vi "SetChannelStatus.vi"(8 "error in (no error)":errorcluster, 10 "Channel Status":string, 11 "Waveform in":waveform(sgl)) -> (0 "error out":errorcluster, 3 "Waveform out":waveform(sgl))   [LabVIEW 2017, in "ChannelStatus.lvlib"]
uses:
  <vilib>/addons/InsightCM/Utilities/ChannelStatus/ChannelStatus.lvlib
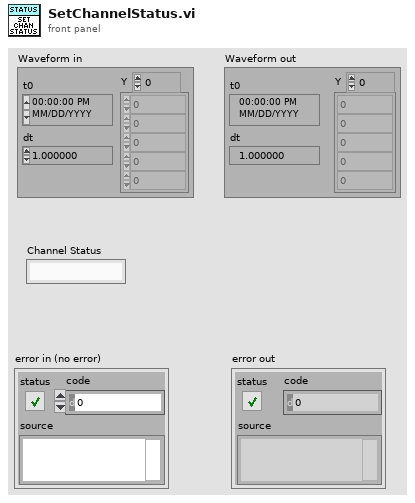
[diagram p1: front panel]
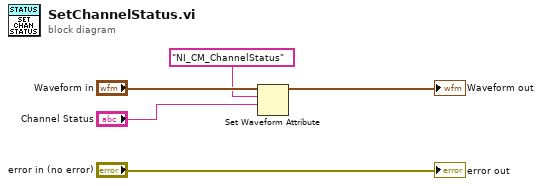
[diagram p0: block diagram]
diagram:
  n1 = Set Waveform Attribute(5:"Channel Status", 6:"NI_CM_ChannelStatus" ("name"), 7:"Waveform in") -> (3:→"Waveform out":waveform(sgl))  [unwired: 1 in, 2 out]
  "error out" <- "error in (no error)"
